vi "Configure Modulation Source.vi"(0 "VISA resource name":refnum<visa-resource-name>, 1 "Internal Waveform (0: Sine)":u16(ring) items=["Sine", "Triangle", "Square", "Ramp", "Noise", "Dual-Sine", "Swept-Sine"], 2 "Modulation Path (1)":u16(ring)=1 items=["1"=1, "2"=2], 3 "Modulation Type (0: Amplitude Modulation)":u16(ring) items=["Amplitude Modulation", "Frequency Modulation", "Phase Modulation"], 5 "Modulation Source (0: Internal1)":u16(ring) items=["Internal1", "Internal2", "External1", "External2"], 7 "Internal Frequency (400 Hz)":dbl=400.0, 9 "Alternate Internal Frequency (400 Hz)":dbl=400.0, 11 "error in (no error)":errorcluster, 12 "External Coupling (1: DC)":u16(ring)=1 items=["AC", "DC"], 13 "External Impedance (0: 50 Ohms)":u16(ring) items=["50 Ohms", "600 Ohms"]) -> (4 "VISA resource name out":refnum<visa-resource-name>, 15 "error out":errorcluster)   [LabVIEW 2011, in "Agilent PSG MXG Series.lvlib"]
doc: "Configures the modulation source and relative parameters of a specific modulation.\n\n<B>Notes:</B>\n(1) This VI is <B>NOT</B> valid in E8247C.\n\n(2) For E8257D, E8267D, N5181A, N5182A, this VI is valid only when the instrument installs <B>Option UNT</B> (AM, FM, phase modulation)."
uses:
  Agilent PSG MXG Series.lvlib
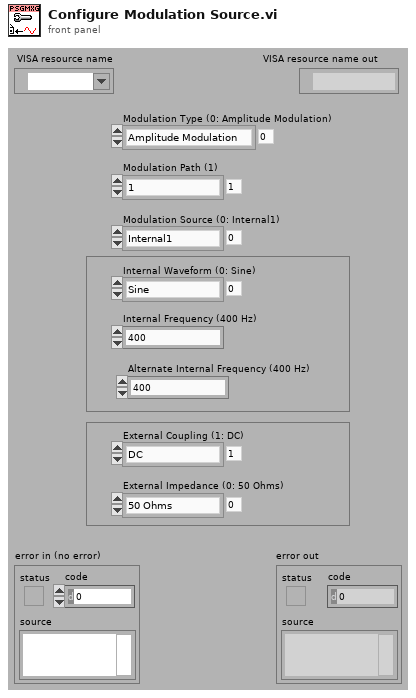
[diagram p1: front panel]
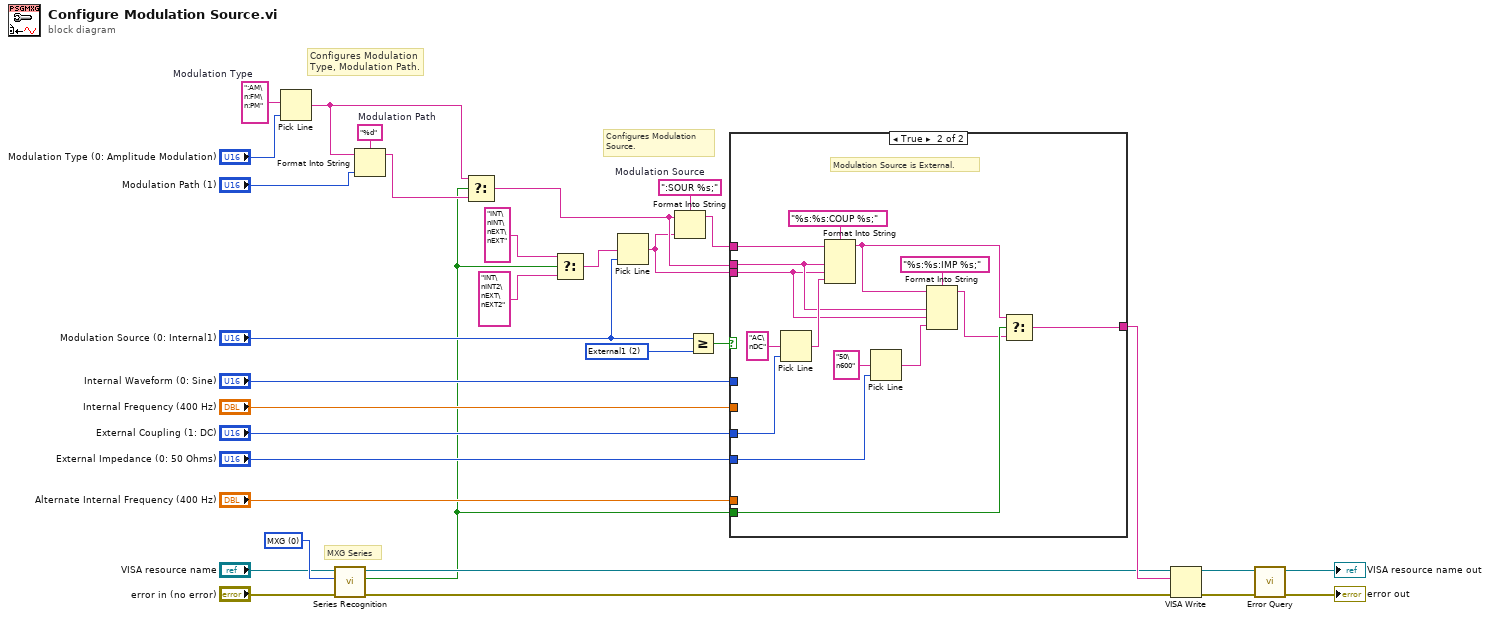
[diagram p0: block diagram]
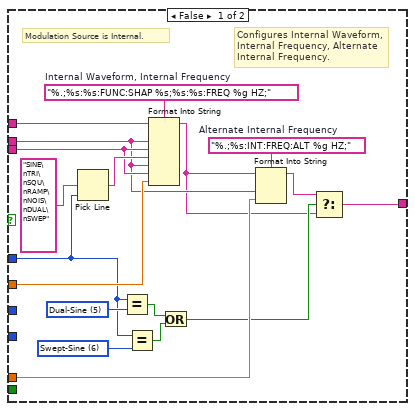
[diagram p2: hidden frame]
diagram:
  w5 = u16 0 items=["MXG", "PSG", "PSG-A", "PSG-C", "PSG-D"] ("Series Type (0: MXG)")
  w25 = u16 2 items=["Internal1", "Internal2", "External1", "External2"] ("Modulation Source (0: Internal1)")
  w26 = ":SOUR %s;"  # Modulation Source
  w29 = "%d"  # Modulation Path
  w32 = ":AM\n:FM\n:PM"  # Modulation Type
  # "Configures Modulation\nSource."
  # "Configures Modulation\nType, Modulation Path."
  # "MXG Series"
  n1 = Pick Line(multi-line string=w32, line index="Modulation Type (0: Amplitude Modulation)") -> (output string=w28:string)  [unwired: 1 in]
  n2 = call "Series Recognition.vi"("error in (no error)"="error in (no error)", "Series Type (0: MXG)"=w5, "VISA resource name"="VISA resource name") -> ("error out"=w8:errorcluster, "Is Series Correct"=w6:bool, "VISA resource name out"=w7:refnum<visa-resource-name>)  [unwired: 6 in]
  n3 = Format Into String(format string=w29, initial string=w28, "Modulation Path (1)") -> (resulting string=w27:string)  [unwired: 1 in, 1 out]
  n4 = Select(t=w28, s=w6, f=w27) -> (s? t:f=w22:string)
  n5 = Select(t="INT\nINT\nEXT\nEXT" ("multi-line string"), s=w6, f="INT\nINT2\nEXT\nEXT2" ("multi-line string")) -> (s? t:f=w16:string)
  n6 = Pick Line(multi-line string=w16, line index="Modulation Source (0: Internal1)") -> (output string=w21:string)  [unwired: 1 in]
  n7 = Format Into String(format string=w26, initial string=w22, w21) -> (resulting string=w9:string)  [unwired: 1 in, 1 out]
  n8 = Greater Or Equal?(x="Modulation Source (0: Internal1)", y=w25) -> (x >= y?=w23:bool)
  n9 = case shown="True" w23 {
    tunnel: w22 -> [w44 w60]
    tunnel: w21 -> [w47 w59]
    tunnel: "Internal Waveform (0: Sine)" -> [w41 _]
    tunnel: "Internal Frequency (400 Hz)" -> [w46 _]
    tunnel: "External Coupling (1: DC)" -> [_ w62]
    tunnel: "External Impedance (0: 50 Ohms)" -> [_ w56]
    tunnel: w6 -> [_ w55]
    tunnel: [w34 w52] -> w11
    tunnel: "Alternate Internal Frequency (400 Hz)" -> [w43 _]
    tunnel: w9 -> [w33 w51]
    frame False {
      w40 = u16 6 items=["Sine", "Triangle", "Square", "Ramp", "Noise", "Dual-Sine", "Swept-Sine"] ("Internal Waveform (0: Sine)")
      w45 = "%.;%s:INT:FREQ:ALT %g HZ;"  # Alternate Internal Frequency
      w42 = u16 5 items=["Sine", "Triangle", "Square", "Ramp", "Noise", "Dual-Sine", "Swept-Sine"] ("Internal Waveform (0: Sine)")
      w50 = "%.;%s:%s:FUNC:SHAP %s;%s:%s:FREQ %g HZ;"  # Internal Waveform, Internal Frequency
      # "Configures Internal Waveform,\nInternal Frequency, Alternate\nInternal Frequency."
      # "Modulation Source is Internal."
      n10 = Pick Line(multi-line string="SINE\nTRI\nSQU\nRAMP\nNOIS\nDUAL\nSWEP", line index=w41) -> (output string=w49:string)  [unwired: 1 in]
      n11 = Equal?(x=w41, y=w42) -> (x = y?=w39:bool)
      n12 = Equal?(x=w41, y=w40) -> (x = y?=w38:bool)
      n13 = Format Into String(format string=w50, initial string=w33, w44, w47, w49, w44, w47, w46) -> (resulting string=w35:string)  [unwired: 1 in, 1 out]
      n14 = Or(x=w39, y=w38) -> (x .or. y?=w37:bool)
      n15 = Format Into String(format string=w45, initial string=w35, w44, w43) -> (resulting string=w36:string)  [unwired: 1 in, 1 out]
      n16 = Select(t=w36, s=w37, f=w35) -> (s? t:f=w34:string)
    }
    frame True {
      # "Modulation Source is External."
      n17 = Pick Line(multi-line string="AC\nDC", line index=w62) -> (output string=w64:string)  [unwired: 1 in]
      n18 = Format Into String(format string="%s:%s:COUP %s;", initial string=w51, w60, w59, w64) -> (resulting string=w54:string)  [unwired: 1 in, 1 out]
      n19 = Pick Line(multi-line string="50\n600", line index=w56) -> (output string=w58:string)  [unwired: 1 in]
      n20 = Format Into String(format string="%s:%s:IMP %s;", initial string=w54, w60, w59, w58) -> (resulting string=w53:string)  [unwired: 1 in, 1 out]
      n21 = Select(t=w54, s=w55, f=w53) -> (s? t:f=w52:string)
    }
  }
  n22 = VISA Write(VISA resource name=w7, write buffer=w11, error in (no error)=w8) -> (VISA resource name out=w13:refnum<visa-resource-name>, error out=w12:errorcluster)  [unwired: 1 out]
  n23 = call "Error Query.vi"("error in (no error)"=w12, "VISA resource name"=w13) -> ("error out"=→"error out":errorcluster, "VISA resource name out"=→"VISA resource name out":refnum<visa-resource-name>)  [unwired: 6 in, 2 out]
